vi "报告存储.vi"(11 "试验时间":timestamp) -> ()   [LabVIEW 2010]
uses:
  全局量/试验配置信息.vi
  全局量/自动测试结果.vi
panel:
  in  "序号":i32
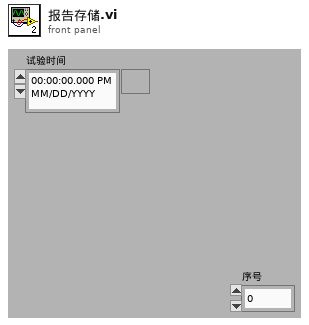
[diagram p1: front panel]
types:
  T1 = cluster{"position (Excel)":cluster{"row":i32, "column":i32}, "name (Excel)":string, "bookmark (Word)":string}
  T2 = cluster{"报告编号":string, "控制板编号":string, "控制板类型":string, "测试人员":string, "测试地点":string, string, u64, "spreadsheet string":string, "spreadsheet string":string, "spreadsheet string":string, "spreadsheet string":string}
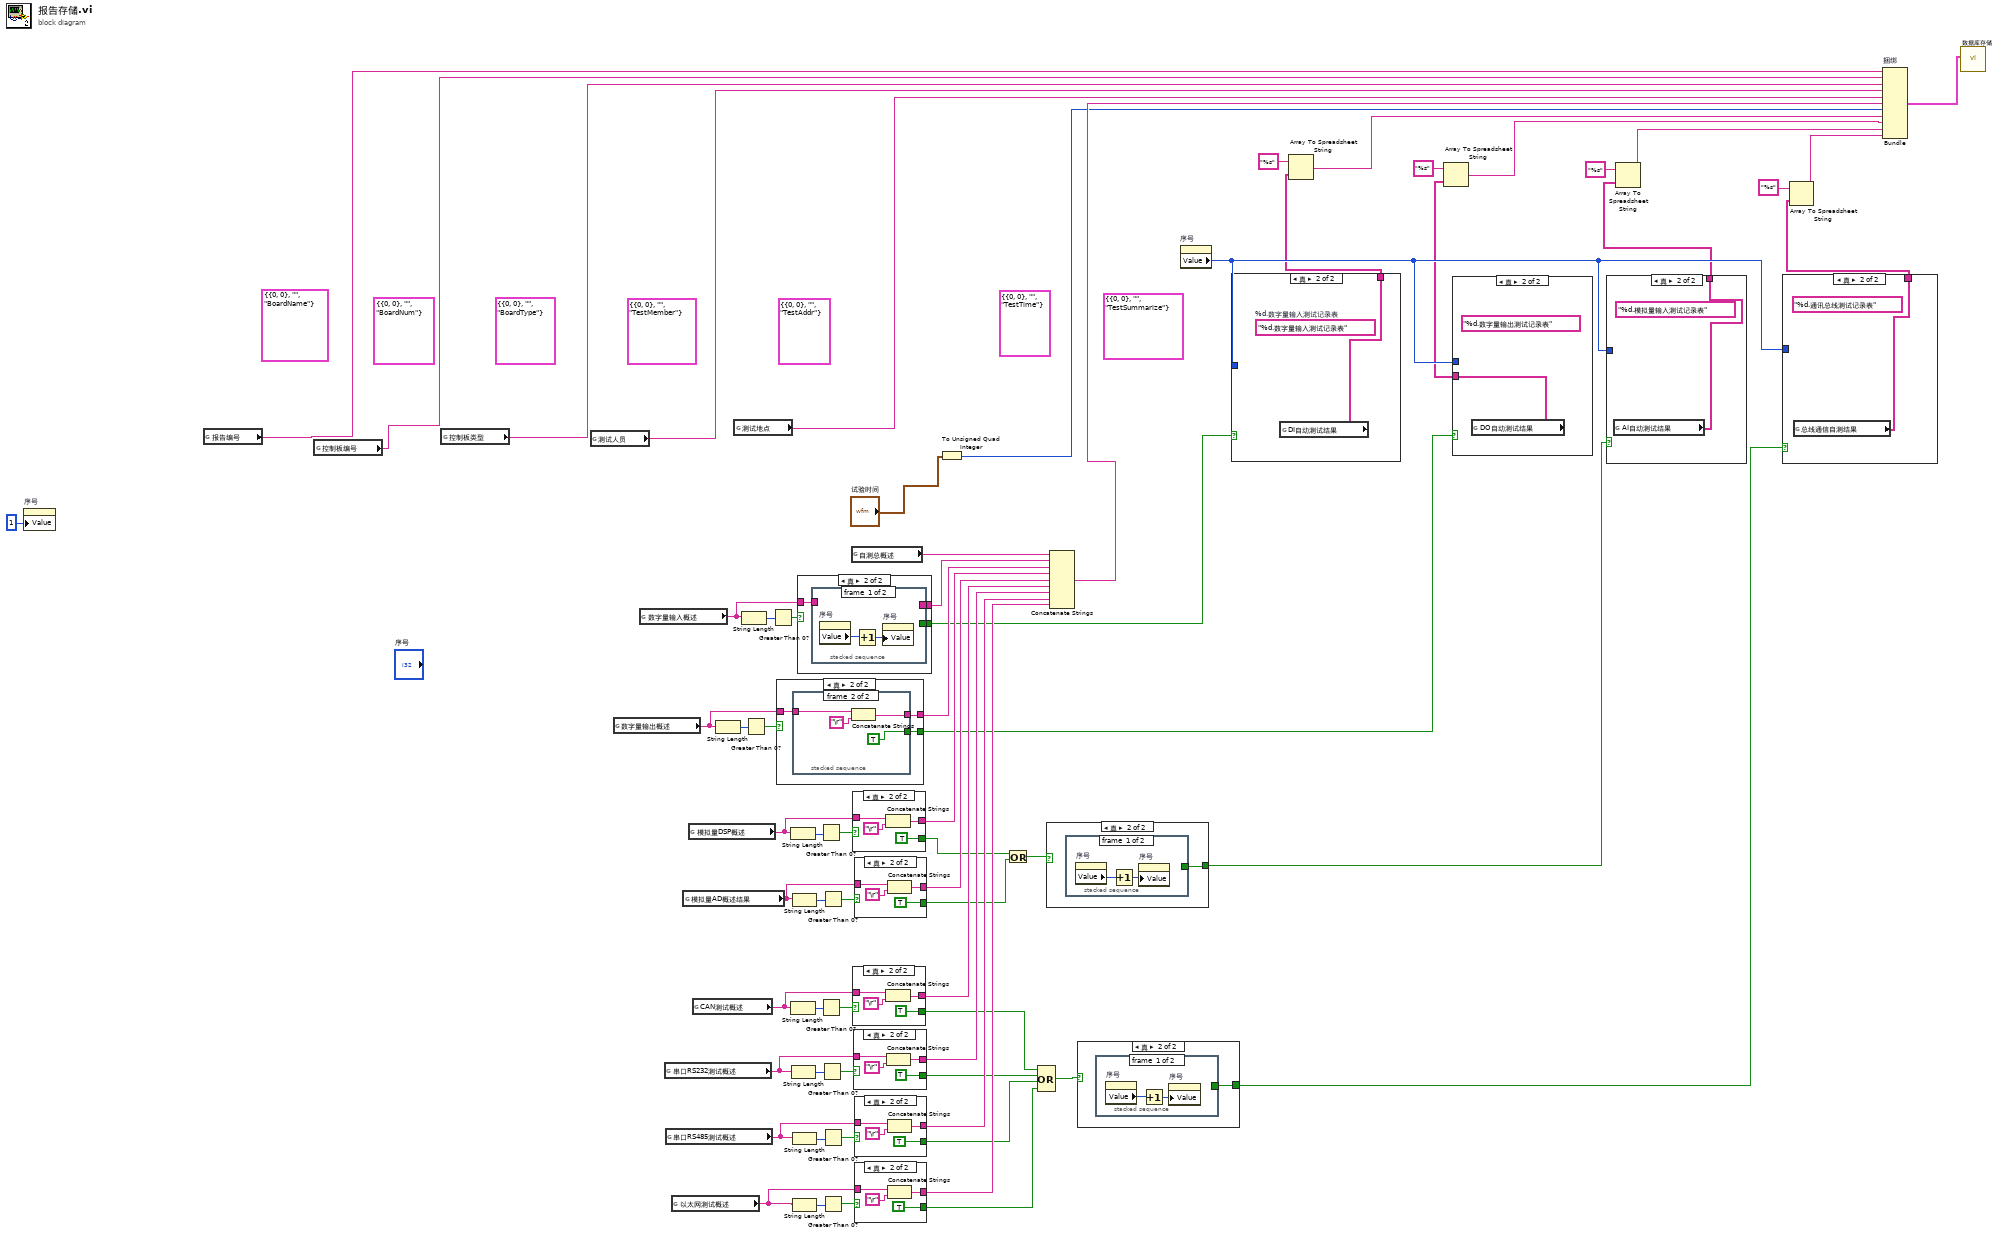
[diagram p0: block diagram]
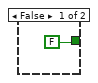
[diagram p2: hidden frame]
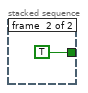
[diagram p3: hidden frame]
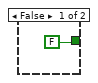
[diagram p4: hidden frame]
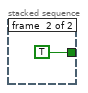
[diagram p5: hidden frame]
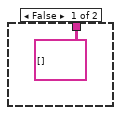
[diagram p6: hidden frame]
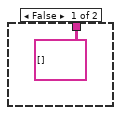
[diagram p7: hidden frame]
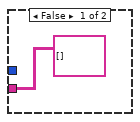
[diagram p8: hidden frame]
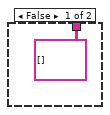
[diagram p9: hidden frame]
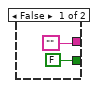
[diagram p10: hidden frame]
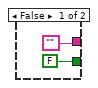
[diagram p11: hidden frame]
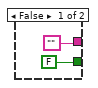
[diagram p12: hidden frame]
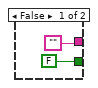
[diagram p13: hidden frame]
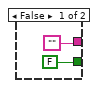
[diagram p14: hidden frame]
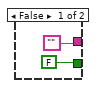
[diagram p15: hidden frame]
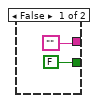
[diagram p16: hidden frame]
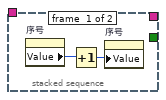
[diagram p17: hidden frame]
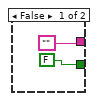
[diagram p18: hidden frame]
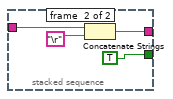
[diagram p19: hidden frame]
diagram:
  (unwired) T1 {"position (Excel)"={"row"=0, "column"=0}, "name (Excel)"="", "bookmark (Word)"="TestSummarize"} ("MS Office parameters")
  (unwired) T1 {"position (Excel)"={"row"=0, "column"=0}, "name (Excel)"="", "bookmark (Word)"="TestAddr"} ("MS Office parameters")
  (unwired) T1 {"position (Excel)"={"row"=0, "column"=0}, "name (Excel)"="", "bookmark (Word)"="TestMember"} ("MS Office parameters")
  (unwired) T1 {"position (Excel)"={"row"=0, "column"=0}, "name (Excel)"="", "bookmark (Word)"="BoardType"} ("MS Office parameters")
  (unwired) T1 {"position (Excel)"={"row"=0, "column"=0}, "name (Excel)"="", "bookmark (Word)"="BoardNum"} ("MS Office parameters")
  (unwired) T1 {"position (Excel)"={"row"=0, "column"=0}, "name (Excel)"="", "bookmark (Word)"="TestTime"} ("MS Office parameters")
  (unwired) T1 {"position (Excel)"={"row"=0, "column"=0}, "name (Excel)"="", "bookmark (Word)"="BoardName"} ("MS Office parameters")
  n1 = property on="序号" class="DigNum (严格)"("Value"=1 ("序号")) -> ()  [unwired: 2 in, 2 out]
  n2 = global read "试验配置信息.vi" "报告编号"() -> (w20:string)
  n3 = global read "试验配置信息.vi" "控制板编号"() -> (w19:string)
  n4 = global read "试验配置信息.vi" "控制板类型"() -> (w18:string)
  n5 = global read "试验配置信息.vi" "测试人员"() -> (w17:string)
  n6 = global read "自动测试结果.vi" "数字量输出概述"() -> (w65:string)
  n7 = global read "自动测试结果.vi" "数字量输入概述"() -> (w66:string)
  n8 = global read "自动测试结果.vi" "串口RS232测试概述"() -> (w53:string)
  n9 = global read "自动测试结果.vi" "串口RS485测试概述"() -> (w48:string)
  n10 = global read "自动测试结果.vi" "以太网测试概述"() -> (w36:string)
  n11 = global read "自动测试结果.vi" "模拟量AD概述结果"() -> (w59:string)
  n12 = global read "自动测试结果.vi" "模拟量DSP概述"() -> (w60:string)
  n13 = global read "自动测试结果.vi" "CAN测试概述"() -> (w54:string)
  n14 = String Length(string=w65) -> (length=w63:i32)
  n15 = global read "试验配置信息.vi" "测试地点"() -> (w16:string)
  n16 = String Length(string=w66) -> (length=w68:i32)
  n17 = Greater Than 0?(x=w63) -> (x > 0?=w64:bool)
  n18 = Greater Than 0?(x=w68) -> (x > 0?=w67:bool)
  n19 = case shown="真" w64 {
    tunnel: w65 -> [_ w73]
    tunnel: ["" w72] -> w44
    tunnel: [FALSE w71] -> w33
    frame False {
    }
    frame True {
      n20 = stacked-sequence {
        tunnel: w73 -> [_ w79]
        tunnel: [_ w77] -> w72
        tunnel: [_ TRUE] -> w71
        frame #0 {
          n21 = property on="序号" class="DigNum (严格)"() -> ("Value"=w75:i32)  [unwired: 2 in, 2 out]
          n22 = Increment(x=w75) -> (x+1=w74:i32)
          n23 = property on="序号" class="DigNum (严格)"("Value"=w74) -> ()  [unwired: 2 in, 2 out]
        }
        frame #1 {
          n24 = Concatenate Strings(w79, "\r") -> (w77:string)
        }
      }
    }
  }
  n25 = String Length(string=w60) -> (length=w62:i32)
  n26 = String Length(string=w54) -> (length=w56:i32)
  n27 = String Length(string=w53) -> (length=w51:i32)
  n28 = String Length(string=w59) -> (length=w57:i32)
  n29 = String Length(string=w48) -> (length=w50:i32)
  n30 = String Length(string=w36) -> (length=w47:i32)
  n31 = case shown="真" w67 {
    tunnel: w66 -> [_ w84]
    tunnel: ["" w83] -> w45
    tunnel: [FALSE w82] -> w34
    frame False {
    }
    frame True {
      n32 = stacked-sequence {
        tunnel: w84 -> [_ w90]
        tunnel: [_ w88] -> w83
        tunnel: [_ TRUE] -> w82
        frame #0 {
          n33 = property on="序号" class="DigNum (严格)"() -> ("Value"=w85:i32)  [unwired: 2 in, 2 out]
          n34 = Increment(x=w85) -> (x+1=w86:i32)
          n35 = property on="序号" class="DigNum (严格)"("Value"=w86) -> ()  [unwired: 2 in, 2 out]
        }
        frame #1 {
          n36 = Concatenate Strings(w90, "\r") -> (w88:string)
        }
      }
    }
  }
  n37 = Greater Than 0?(x=w62) -> (x > 0?=w61:bool)
  n38 = Greater Than 0?(x=w56) -> (x > 0?=w55:bool)
  n39 = Greater Than 0?(x=w51) -> (x > 0?=w52:bool)
  n40 = Greater Than 0?(x=w57) -> (x > 0?=w58:bool)
  n41 = Greater Than 0?(x=w50) -> (x > 0?=w49:bool)
  n42 = Greater Than 0?(x=w47) -> (x > 0?=w37:bool)
  n43 = global read "自动测试结果.vi" "自测总概述"() -> (w46:string)
  n44 = case shown="真" w61 {
    tunnel: w60 -> [_ w96]
    tunnel: ["" w94] -> w43
    tunnel: [FALSE TRUE] -> w32
    frame False {
    }
    frame True {
      n45 = Concatenate Strings(w96, "\r") -> (w94:string)
    }
  }
  n46 = case shown="真" w55 {
    tunnel: w54 -> [_ w102]
    tunnel: ["" w100] -> w41
    tunnel: [FALSE TRUE] -> w29
    frame False {
    }
    frame True {
      n47 = Concatenate Strings(w102, "\r") -> (w100:string)
    }
  }
  n48 = case shown="真" w52 {
    tunnel: w53 -> [_ w108]
    tunnel: ["" w106] -> w40
    tunnel: [FALSE TRUE] -> w28
    frame False {
    }
    frame True {
      n49 = Concatenate Strings(w108, "\r") -> (w106:string)
    }
  }
  n50 = case shown="真" w58 {
    tunnel: w59 -> [_ w114]
    tunnel: ["" w112] -> w42
    tunnel: [FALSE TRUE] -> w31
    frame False {
    }
    frame True {
      n51 = Concatenate Strings(w114, "\r") -> (w112:string)
    }
  }
  n52 = case shown="真" w49 {
    tunnel: w48 -> [_ w120]
    tunnel: ["" w118] -> w39
    tunnel: [FALSE TRUE] -> w27
    frame False {
    }
    frame True {
      n53 = Concatenate Strings(w120, "\r") -> (w118:string)
    }
  }
  n54 = case shown="真" w37 {
    tunnel: w36 -> [_ w126]
    tunnel: ["" w124] -> w38
    tunnel: [FALSE TRUE] -> w26
    frame False {
    }
    frame True {
      n55 = Concatenate Strings(w126, "\r") -> (w124:string)
    }
  }
  n56 = To Unsigned Quad Integer(1:"试验时间") -> (0:w14:u64)
  n57 = Or(x=w32, y=w31) -> (x .or. y?=w30:bool)
  n58 = Compound Arithmetic op=OR(w29, w28, w27, w26) -> (w25:bool)
  n59 = case shown="真" w30 {
    tunnel: [FALSE w128] -> w24
    frame False {
    }
    frame True {
      n60 = stacked-sequence {
        tunnel: [_ TRUE] -> w128
        frame #0 {
          n61 = property on="序号" class="DigNum (严格)"() -> ("Value"=w130:i32)  [unwired: 2 in, 2 out]
          n62 = Increment(x=w130) -> (x+1=w129:i32)
          n63 = property on="序号" class="DigNum (严格)"("Value"=w129) -> ()  [unwired: 2 in, 2 out]
        }
        frame #1 {
        }
      }
    }
  }
  n64 = Concatenate Strings(w46, w45, w44, w43, w42, w41, w40, w39, w38) -> (w15:string)
  n65 = case shown="真" w25 {
    tunnel: [FALSE w133] -> w22
    frame False {
    }
    frame True {
      n66 = stacked-sequence {
        tunnel: [_ TRUE] -> w133
        frame #0 {
          n67 = property on="序号" class="DigNum (严格)"() -> ("Value"=w135:i32)  [unwired: 2 in, 2 out]
          n68 = Increment(x=w135) -> (x+1=w134:i32)
          n69 = property on="序号" class="DigNum (严格)"("Value"=w134) -> ()  [unwired: 2 in, 2 out]
        }
        frame #1 {
        }
      }
    }
  }
  n70 = property on="序号" class="DigNum (严格)"() -> ("Value"=w23:i32)  [unwired: 2 in, 2 out]
  n71 = case shown="真" w34 {
    tunnel: w23 -> [_ _]
    tunnel: [string[][] [] ("DI自动测试结果") w138] -> w12
    frame False {
    }
    frame True {
      (unwired) "%d.数字量输入测试记录表"  # %d.数字量输入测试记录表
      n72 = global read "自动测试结果.vi" "DI自动测试结果"() -> (w138:string[][])
    }
  }
  n73 = Array To Spreadsheet String(array=w12, 3:"%s" ("格式字符串")) -> (spreadsheet string=w11:string)  [unwired: 1 in]
  n74 = case shown="真" w33 {
    tunnel: w23 -> [_ _]
    tunnel: [string[][] [] ("DO自动测试结果") w140] -> w9
    frame False {
    }
    frame True {
      (unwired) "%d.数字量输出测试记录表"
      n75 = global read "自动测试结果.vi" "DO自动测试结果"() -> (w140:string[][])
    }
  }
  n76 = Array To Spreadsheet String(array=w9, 3:"%s" ("格式字符串")) -> (spreadsheet string=w8:string)  [unwired: 1 in]
  n77 = case shown="真" w24 {
    tunnel: w23 -> [_ _]
    tunnel: [string[][] [] ("AI自动测试结果") w142] -> w6
    frame False {
    }
    frame True {
      (unwired) "%d.模拟量输入测试记录表"
      n78 = global read "自动测试结果.vi" "AI自动测试结果"() -> (w142:string[][])
    }
  }
  n79 = Array To Spreadsheet String(array=w6, 3:"%s" ("格式字符串")) -> (spreadsheet string=w5:string)  [unwired: 1 in]
  n80 = case shown="真" w22 {
    tunnel: w23 -> [_ _]
    tunnel: [string[][] [] ("总线通信自测结果") w144] -> w3
    frame False {
    }
    frame True {
      (unwired) "%d.通讯总线测试记录表"
      n81 = global read "自动测试结果.vi" "总线通信自测结果"() -> (w144:string[][])
    }
  }
  n82 = Array To Spreadsheet String(array=w3, 3:"%s" ("格式字符串")) -> (spreadsheet string=w2:string)  [unwired: 1 in]
  n83 = Bundle "捆绑"("报告编号"=w20, "控制板编号"=w19, "控制板类型"=w18, "测试人员"=w17, "测试地点"=w16, w15, w14, "spreadsheet string"=w11, "spreadsheet string"=w8, "spreadsheet string"=w5, "spreadsheet string"=w2) -> (w1:T2)  [unwired: 1 in]
  n84 = call "数据库存储.vi"("输出簇 2"=w1) -> ()  [unwired: 10 in]
